vi "Read Read Mode.vi"(8 "error in (no error)":errorcluster, 11 "TCPConnection in":refnum<class "LocalQueueConnection.lvclass">) -> (0 "error out":errorcluster, 2 "Read Mode":T1(ring)=enum."Immediate", 3 "TCPConnection out":refnum<class "LocalQueueConnection.lvclass">)   [LabVIEW 2013, in "MQTT_Queue.lvlib" / "LocalQueueConnection.lvclass"]
uses:
  LocalQueueConnection.lvclass
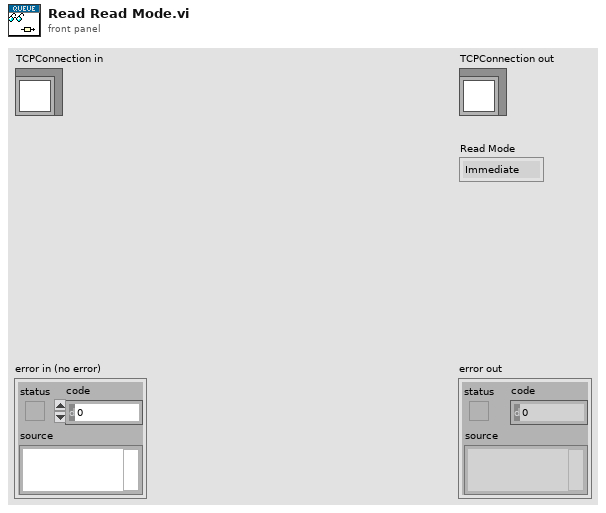
[diagram p1: front panel]
types:
  T1 = enum16{"Standard", "Buffered", "CRLF", "Immediate"}
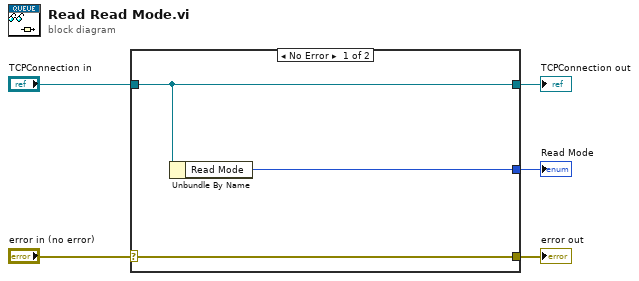
[diagram p0: block diagram]
diagram:
  n1 = case shown="No Error" "error in (no error)" {
    selector: "error in (no error)" -> [w8 w9]
    tunnel: [w8 w9] -> w4
    tunnel: [w7 w10] -> w2
    tunnel: "TCPConnection in" -> [w7 w10]
    tunnel: [w6 _] -> w1
    frame No Error {
      n2 = Unbundle By Name(w7) -> ("Read Mode"=w6:T1)
    }
    frame Error {
    }
  }
  "error out" <- w4
  "TCPConnection out" <- w2
  "Read Mode" <- w1
